vi "Get Data.vi"(6 "Iteration":i32, 8 "error in":errorcluster, 9 "N_DataSets\nper Gen5":i32=16, 10 "Device Count":i32, 11 "N_Channels\nper Dataset (NCD)":i32=8) -> (0 "error out":errorcluster, 2 "Data out":sgl[](array[numeric]))   [LabVIEW 2015, in "G 5.lvlib"]
uses:
  G 5.lvlib
  AMTIUSBDevice.dll
panel:
  in  "stop 3":bool
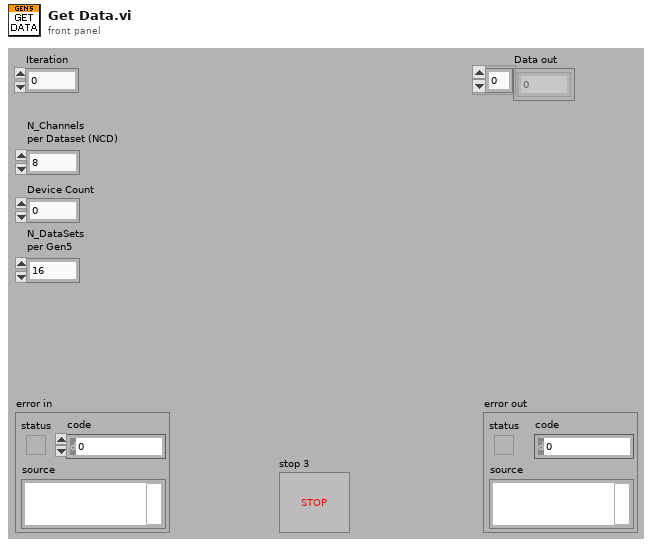
[diagram p1: front panel]
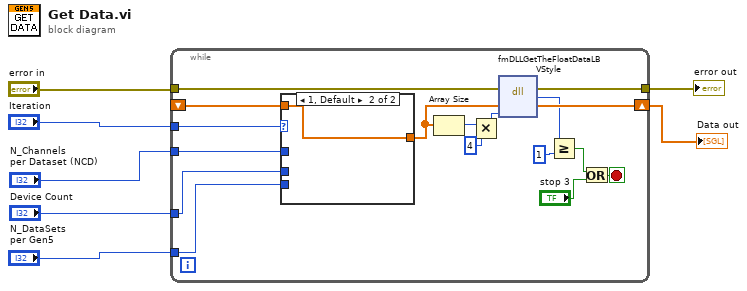
[diagram p0: block diagram]
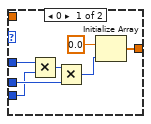
[diagram p2: hidden frame]
diagram:
  n1 = while {
    tunnel: "error in" -> [w24]
    tunnel: [w23] -> w5
    shift-right: [w22] -> w6
    shift-left: _ -> [w12]
    tunnel: "Iteration" -> [w16]
    tunnel: "N_Channels\nper Dataset (NCD)" -> [w10]
    tunnel: "Device Count" -> [w9]
    tunnel: "N_DataSets\nper Gen5" -> [w8]
    stop <- w19 stop-if-true
    n2 = case shown="1, Default" w16 {
      tunnel: [w28 w32] -> w11
      tunnel: w12 -> [_ w32]
      tunnel: w10 -> [w27 _]
      tunnel: w9 -> [w26 _]
      tunnel: w8 -> [w25 _]
      frame 0 {
        n3 = Multiply(x=w27, y=w25) -> (x*y=w30:i32)
        n4 = Multiply(x=w30, y=w26) -> (x*y=w29:i32)
        n5 = Initialize Array(0.0 ("element"), w29) -> (w28:dbl[])
      }
      frame 1, Default {
      }
    }
    n6 = Array Size(array=w11) -> (size(s)=w14:i32)
    n7 = Multiply(x=w14, y=4) -> (x*y=w13:i32)
    n8 = dll-call lib="AMTIUSBDevice.dll" fn="fmDLLGetTheFloatDataLBVStyle"(error in=w24, "data"=w11, "size"=w13) -> (error out=w23:errorcluster, "LV data"=w17:i32, "data"=w22:sgl[])  [unwired: 3 in, 1 out]
    n9 = Greater Or Equal?(x=w17, y=1) -> (x >= y?=w21:bool)
    n10 = Or(x=w21, y="stop 3") -> (x .or. y?=w19:bool)
  }
  "Data out" <- w6
  "error out" <- w5
